vi "ProcessControl-Stop.vi"(2 "PROCESS":string, 9 "error in (no error)":errorcluster) -> (6 "error out":errorcluster)   [LabVIEW 2009]
uses:
  ProcessControl.ctl
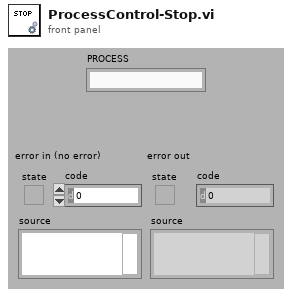
[diagram p1: front panel]
types:
  T1 = typedef "ProcessControl.ctl" = enum16{"STOP"}
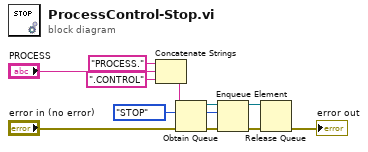
[diagram p0: block diagram]
diagram:
  w5 = ProcessControl."STOP" ("ProcessControl")
  n1 = Concatenate Strings("PROCESS." ("chaîne"), "PROCESS", ".CONTROL" ("chaîne")) -> (w11:string)
  n2 = Obtain Queue(name (unnamed)=w11, element data type=w5, error in (no error)="error in (no error)") -> (queue out=w6:refnum<queue>, error out=w7:errorcluster)  [unwired: 2 in, 1 out]
  n3 = Enqueue Element(queue=w6, element=w5, error in (no error)=w7) -> (queue out=w3:refnum<queue>, error out=w4:errorcluster)  [unwired: 2 out]
  n4 = Release Queue(queue=w3, error in (no error)=w4) -> (error out=→"error out":errorcluster)  [unwired: 3 out]
